vi "bats.parser.vi"(10 "data_valid":bool, 11 "data":u8) -> (1 "tlast":bool, 2 "tvalid":bool, 3 "tdata":u8)   [LabVIEW 2020]
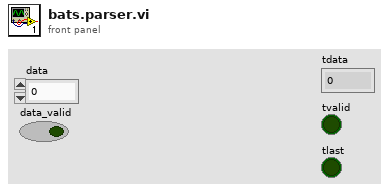
[diagram p1: front panel]
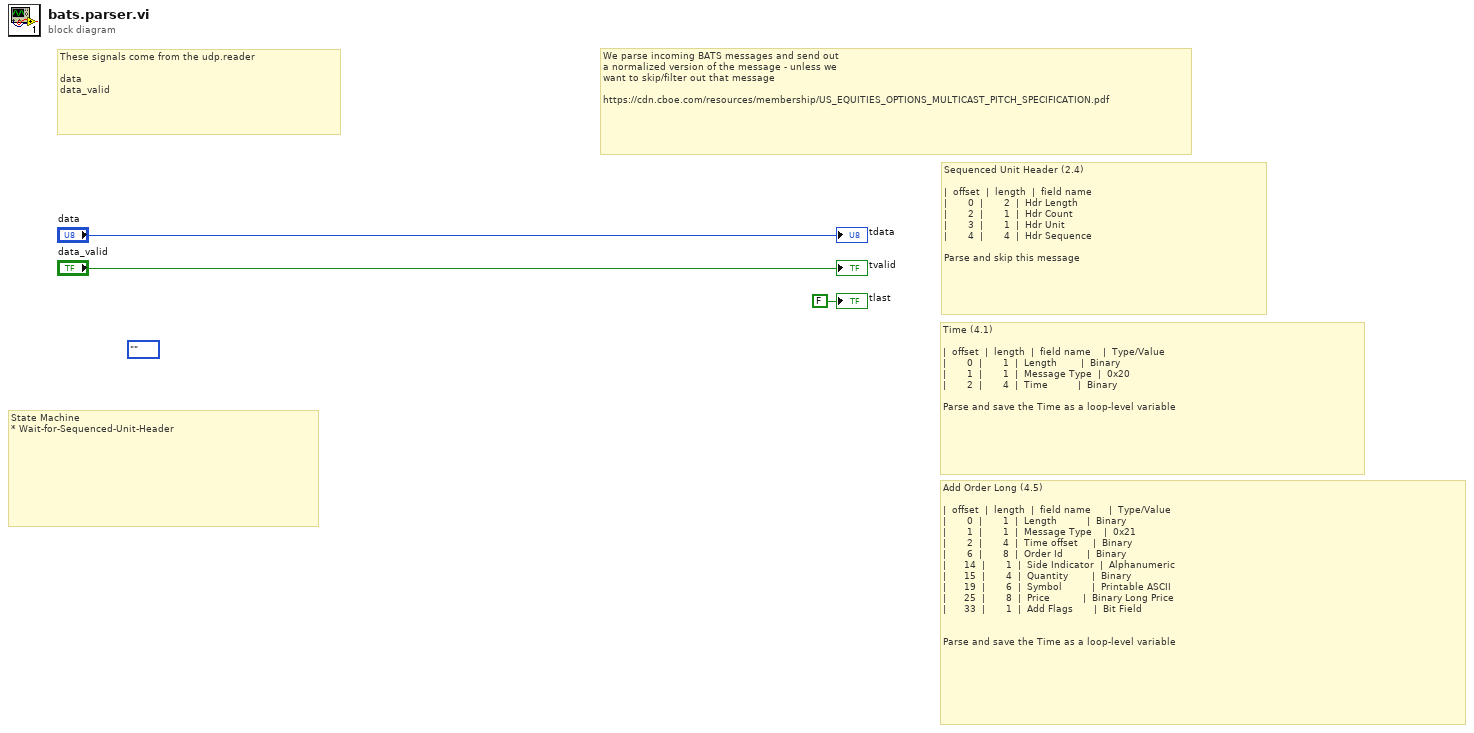
[diagram p0: block diagram]
diagram:
  (unwired) enum16{""}.""
  # "Add Order Long (4.5)\n\n|  offset  |  length  |  field name      |  Type/Value\n|       0  |       1  |  Length          |  Binary\n|       1  |       1  |  Message Type    |  0x21\n|       2  |       4  |  Time offset     |  Binary\n|       6  |       8  |  Order Id        |  Binary\n|      14  |       1  |  Side Indicator  |  Alphanumeric\n|      15  |       4  |  Quantity        |  Binary\n|      19  |       6  |  Symbol          |  Printable ASCII\n|      25  |       8  |  Price           |  Binary Long Price\n|      33  |       1  |  Add Flags       |  Bit Field\n\n\nParse and save the Time as a loop-level variable"
  # "Time (4.1)\n\n|  offset  |  length  |  field name    |  Type/Value\n|       0  |       1  |  Length        |  Binary\n|       1  |       1  |  Message Type  |  0x20\n|       2  |       4  |  Time          |  Binary\n\nParse and save the Time as a loop-level variable"
  # "Sequenced Unit Header (2.4)\n\n|  offset  |  length  |  field name\n|       0  |       2  |  Hdr Length\n|       2  |       1  |  Hdr Count\n|       3  |       1  |  Hdr Unit\n|       4  |       4  |  Hdr Sequence\n\nParse and skip this message"
  # "State Machine\n* Wait-for-Sequenced-Unit-Header"
  # "We parse incoming BATS messages and send out\na normalized version of the message - unless we\nwant to skip/filter out that message\n\nhttps://cdn.cboe.com/resources/membership/US_EQUITIES_OPTIONS_MULTICAST_PITCH_SPECIFICATION.pdf"
  # "These signals come from the udp.reader\n\ndata\ndata_valid"
  "tdata" <- "data"
  "tvalid" <- "data_valid"
  "tlast" <- FALSE ("tlast")
